vi "solar_addon.vi"(7 "Action (Launch)":enum8{"Launch", "Initialize", "Shutdown"}(ring), 8 "error in (no error)":errorcluster, 9 "SOLAR Refnum":T1, 10 "AddonVIs (Initialize only)":refnum<vi>[](array[refnum]), 11 "Launch Addon VI":string) -> (0 "error out":errorcluster, 3 "Addons (vi,title)":string[][](array[string]))   [LabVIEW 2018]
doc: "This handles the Addon VIs."
uses:
  solar/solar_ctl SOLAR Refnum.ctl
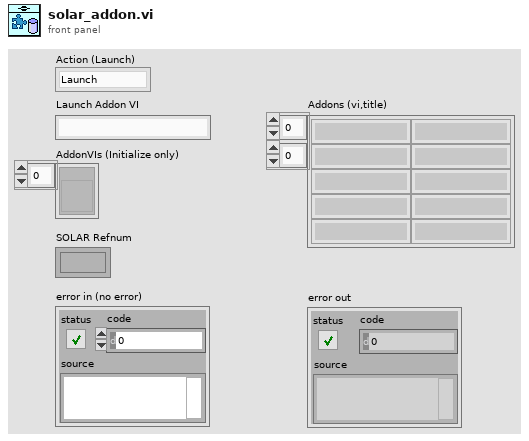
[diagram p1: front panel]
types:
  T1 = typedef "solar_ctl SOLAR Refnum.ctl" = refnum<k1>
  T2 = cluster{"VIName":string, "Title":string, "VI Refnum":refnum<vi>, "Exit":refnum<user-event>}[]
  T3 = cluster{"VIName":string, "Title":string, "VI Refnum":refnum<vi>, "Exit":refnum<user-event>}
  T4 = enum32{"Invalid", "Standard", "Closed", "Hidden", "Minimized", "Maximized"}
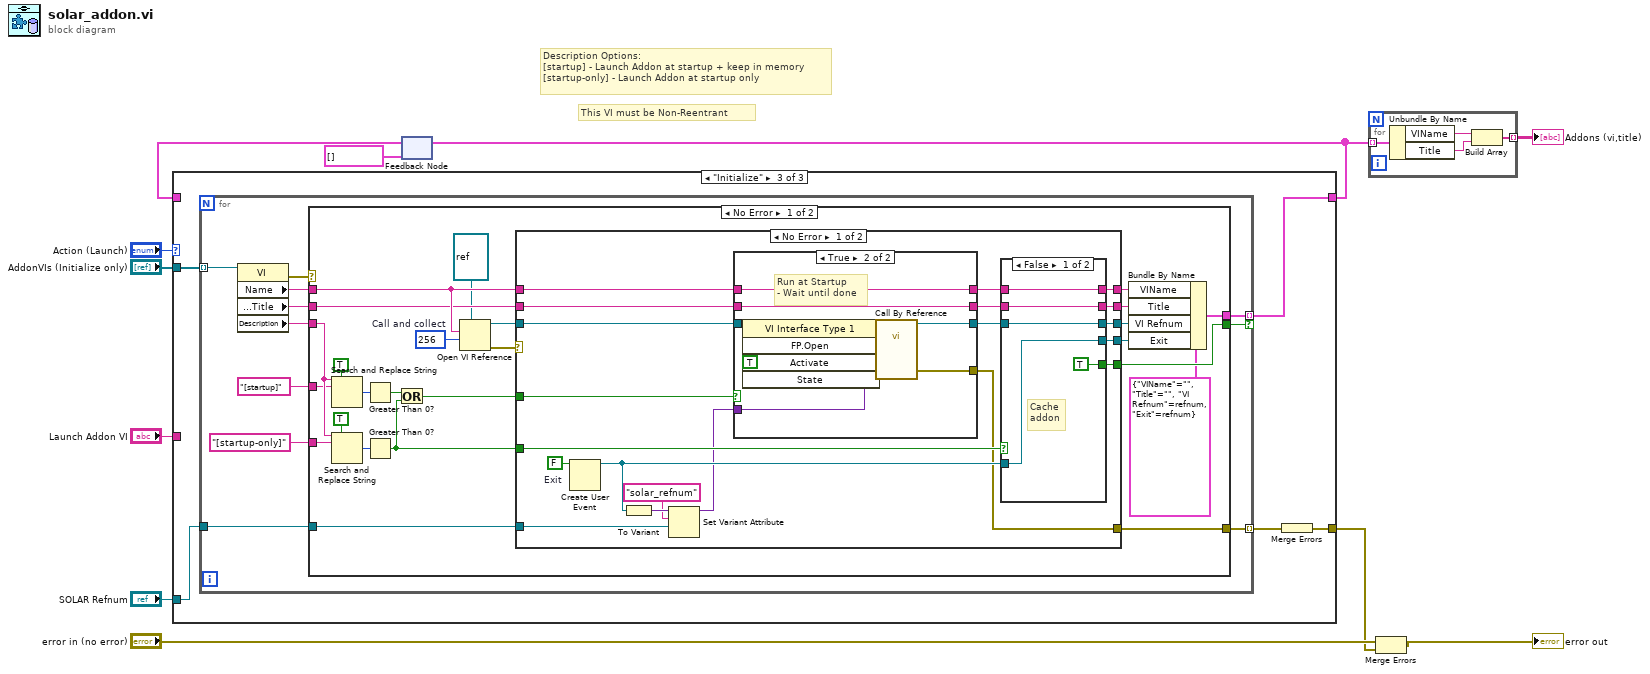
[diagram p0: block diagram]
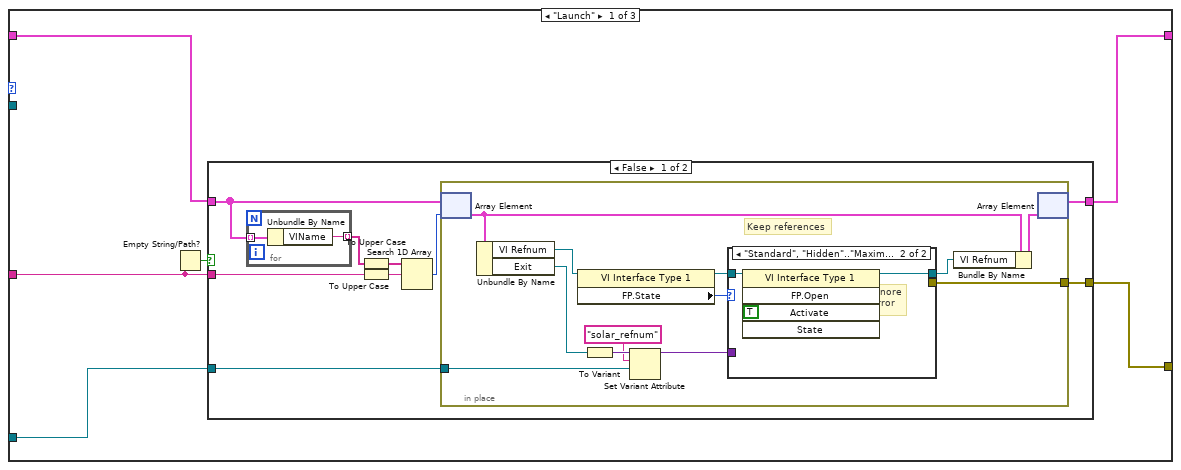
[diagram p2: hidden frame]
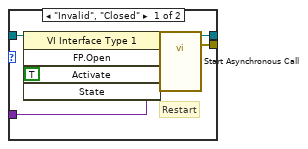
[diagram p3: hidden frame]
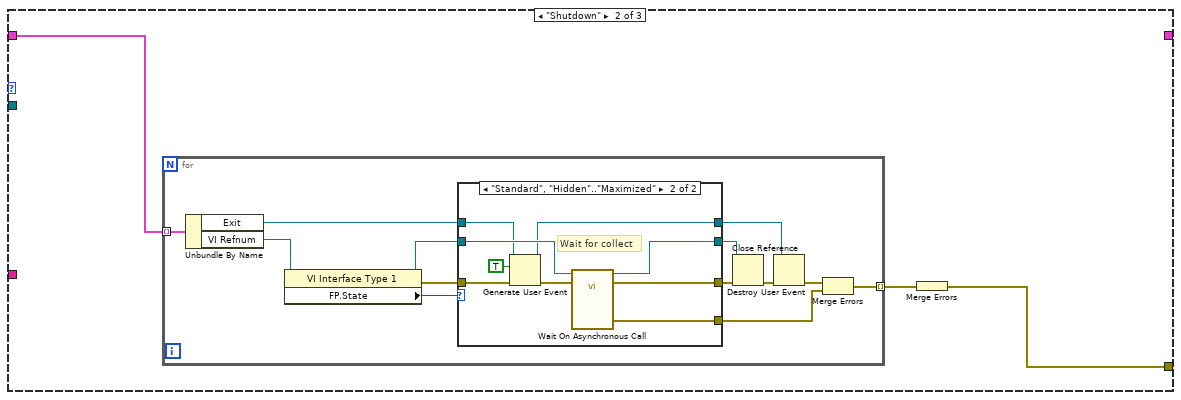
[diagram p5: hidden frame]
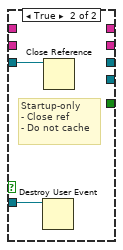
[diagram p7: hidden frame]
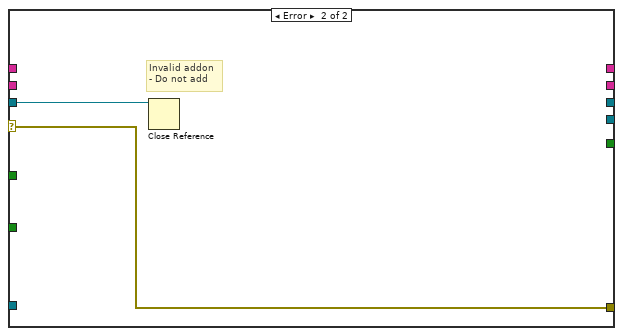
[diagram p9: hidden frame]
diagram:
  # "Description Options:\n[startup] - Launch Addon at startup + keep in memory\n[startup-only] - Launch Addon at startup only"
  # "This VI must be Non-Reentrant"
  n1 = feedback #1(T2 [] ("Array 2")) -> (w4:T2)
  n2 = case shown="\"Initialize\"" "Action (Launch)" {
    tunnel: "AddonVIs (Initialize only)" -> [_ _ w83]
    tunnel: "Launch Addon VI" -> [w17 _ _]
    tunnel: [w13 _ w82] -> w2
    tunnel: w4 -> [w14 w53 _]
    tunnel: "SOLAR Refnum" -> [w12 _ w81]
    tunnel: [w15 w51 w79] -> w3
    frame "Launch" {
      n3 = Empty String/Path?(string/path=w17) -> (empty?=w16:bool)
      n4 = case shown="False" w16 {
        tunnel: w17 -> [w25 _]
        tunnel: w14 -> [w21 w50]
        tunnel: [w22 _] -> w15
        tunnel: [w19 w50] -> w13
        tunnel: w12 -> [w18 _]
        frame False {
          n5 = for {
            tunnel: w21 -> [w49] mode=indexing
            tunnel: [w48] -> w23 mode=indexing
            n6 = Unbundle By Name(w49) -> ("VIName"=w48:string)
          }
          n7 = To Upper Case(1:w23) -> (0:w26:string[])
          n8 = To Upper Case(1:w25) -> (0:w24:string)
          n9 = Search 1D Array(1D array=w26, element=w24) -> (index of element=w20:i32)  [unwired: 1 in]
          n10 = in-place {
            in-place-border: [w38] -> w22
            in-place-border: w18 -> [w29]
            # "Keep references"
            n11 = in-place-array #2(w21, w20) -> (w37:T3)
            n12 = Unbundle By Name(w37) -> ("VI Refnum"=w34:refnum<vi>, "Exit"=w30:refnum<user-event>)
            n13 = property class="VI Interface Type 1"(reference=w34) -> (reference out=w33:refnum<vi>, "FP.State"=w27:T4)  [unwired: 1 in, 1 out]
            n14 = To Variant(anything=w30) -> (Variant=w32:variant)
            n15 = Set Variant Attribute(Variant=w32, name="solar_refnum", value=w29) -> (Variant out=w28:variant)  [unwired: 1 in, 2 out]
            n16 = case shown="\"Standard\", \"Hidden\"..\"Maximized\"" w27 {
              tunnel: [w44 _] -> w38
              tunnel: [w43 w45] -> w35
              tunnel: w33 -> [w41 w46]
              tunnel: w28 -> [w39 _]
              frame "Invalid", "Closed" {
                # "Restart"
                n17 = invoke class="VI Interface Type 1" method="FP.Open"(reference=w41, "Activate"=TRUE ("Activate?")) -> (reference out=w40:refnum<vi>)  [unwired: 3 in, 4 out]
                n18 = call-by-ref "Start Asynchronous Call"(reference=w40, "Variant"=w39) -> (reference out=w43:refnum<vi>, error out=w44:errorcluster)  [unwired: 11 in, 1 out]
              }
              frame "Standard", "Hidden".."Maximized" {
                # "Ignore\nerror"
                n19 = invoke class="VI Interface Type 1" method="FP.Open"(reference=w46, "Activate"=TRUE ("Activate?")) -> (reference out=w45:refnum<vi>)  [unwired: 3 in, 4 out]
              }
            }
            n20 = Bundle By Name(cluster=w37, "VI Refnum"=w35) -> (w36:T3)
            n21 = in-place-array #2(w36) -> (w19:T2)  [unwired: 1 out]
          }
        }
        frame True {
          # "Do nothing"
        }
      }
    }
    frame "Shutdown" {
      n22 = for {
        tunnel: w53 -> [w66] mode=indexing
        tunnel: [w55] -> w52 mode=indexing
        n23 = Unbundle By Name(w66) -> ("Exit"=w63:refnum<user-event>, "VI Refnum"=w62:refnum<vi>)
        n24 = property class="VI Interface Type 1"(reference=w62) -> (reference out=w65:refnum<vi>, error out=w61:errorcluster, "FP.State"=w64:T4)  [unwired: 1 in]
        n25 = case shown="\"Standard\", \"Hidden\"..\"Maximized\"" w64 {
          tunnel: w61 -> [w69 w76]
          tunnel: w65 -> [w68 w78]
          tunnel: w63 -> [w67 w75]
          tunnel: [w69 w72] -> w59
          tunnel: [w68 w73] -> w58
          tunnel: [w67 w71] -> w57
          tunnel: [_ w70] -> w54
          frame "Invalid", "Closed" {
          }
          frame "Standard", "Hidden".."Maximized" {
            # "Wait for collect"
            n26 = Generate User Event(user event=w75, event data cluster=TRUE ("event data"), error in=w76) -> (user event out=w71:refnum<user-event>, error out=w74:errorcluster)  [unwired: 1 in]
            n27 = call-by-ref "Wait On Asynchronous Call"(reference=w78, error in=w74) -> (reference out=w73:refnum<vi>, error out=w72:errorcluster, 0:"error out"=w70:errorcluster)  [unwired: 11 in]
          }
        }
        n28 = Close Reference(reference=w58, error in (no error)=w59) -> (error out=w60:errorcluster)
        n29 = Destroy User Event(user event=w57, error in=w60) -> (error out=w56:errorcluster)
        n30 = Merge Errors(w56, w54) -> (w55:errorcluster)
      }
      n31 = Merge Errors(w52) -> (w51:errorcluster)
    }
    frame "Initialize" {
      n32 = for {
        tunnel: w83 -> [w94] mode=indexing
        tunnel: [w90] -> w82 mode=indexing if=w89
        tunnel: w81 -> [w85]
        tunnel: [w84] -> w80 mode=indexing
        n33 = property class="VI"(reference=w94) -> (error out=w88:errorcluster, "Name"=w92:string, "Front Panel.Title"=w91:string, "Description"=w93:string)  [unwired: 1 in, 1 out]
        n34 = case shown="No Error" w88 {
          selector: w88 -> [_ w160]
          tunnel: w93 -> [w115 _]
          tunnel: w92 -> [w113 _]
          tunnel: w91 -> [w112 _]
          tunnel: [w104 _] -> w90
          tunnel: [w106 _] -> w89
          tunnel: "[startup]" ("search string") -> [w109 _]
          tunnel: "[startup-only]" ("search string") -> [w108 _]
          tunnel: w85 -> [w98 _]
          tunnel: [w95 w160] -> w84
          frame No Error {
            w114 = 256  # Call and collect
            n35 = Search and Replace String(replace all?=TRUE ("replace all? (F)"), input string=w115, search string=w109) -> (number of replacements=w117:i32)  [unwired: 5 in, 3 out]
            n36 = Search and Replace String(replace all?=TRUE ("replace all? (F)"), input string=w115, search string=w108) -> (number of replacements=w118:i32)  [unwired: 5 in, 3 out]
            n37 = Greater Than 0?(x=w117) -> (x > 0?=w110:bool)
            n38 = Greater Than 0?(x=w118) -> (x > 0?=w100:bool)
            n39 = Or(x=w110, y=w100) -> (x .or. y?=w105:bool)
            n40 = Open VI Reference(type specifier VI Refnum (for type only)=refnum<vi> refnum, vi path=w113, options=w114) -> (vi reference=w111:refnum<vi>, error out=w107:errorcluster)  [unwired: 3 in]
            n41 = case shown="No Error" w107 {
              selector: w107 -> [_ w158]
              tunnel: w113 -> [w138 _]
              tunnel: w112 -> [w137 _]
              tunnel: w111 -> [w122 w159]
              tunnel: [w129 _] -> w106
              tunnel: w105 -> [w139 _]
              tunnel: [w135 _] -> w103
              tunnel: [w133 _] -> w102
              tunnel: [w131 _] -> w101
              tunnel: w100 -> [w136 _]
              tunnel: w98 -> [w125 _]
              tunnel: [w123 _] -> w96
              tunnel: [w120 w158] -> w95
              frame No Error {
                w128 = FALSE  # Exit
                n42 = Create User Event(user event datatype=w128) -> (user event=w124:refnum<user-event>)  [unwired: 1 in, 1 out]
                n43 = To Variant(anything=w124) -> (Variant=w127:variant)
                n44 = Set Variant Attribute(Variant=w127, name="solar_refnum", value=w125) -> (Variant out=w121:variant)  [unwired: 1 in, 2 out]
                n45 = case shown="True" w139 {
                  tunnel: w122 -> [w147 w156]
                  tunnel: [w147 w152] -> w130
                  tunnel: [w149 w155] -> w134
                  tunnel: w138 -> [w149 w155]
                  tunnel: w137 -> [w148 w154]
                  tunnel: [w148 w154] -> w132
                  tunnel: w121 -> [_ w151]
                  tunnel: [_ w150] -> w120
                  frame False {
                  }
                  frame True {
                    # "Run at Startup\n- Wait until done"
                    n46 = invoke class="VI Interface Type 1" method="FP.Open"(reference=w156, "Activate"=TRUE ("Activate?")) -> (reference out=w153:refnum<vi>)  [unwired: 3 in, 4 out]
                    n47 = call-by-ref "?"(reference=w153, "Variant"=w151) -> (reference out=w152:refnum<vi>, "error out"=w150:errorcluster)  [unwired: 11 in, 1 out]
                  }
                }
                n48 = case shown="False" w136 {
                  tunnel: [w144 _] -> w135
                  tunnel: w134 -> [w144 _]
                  tunnel: [w143 _] -> w133
                  tunnel: w132 -> [w143 _]
                  tunnel: [w142 _] -> w131
                  tunnel: w130 -> [w142 w146]
                  tunnel: [TRUE _] -> w129
                  tunnel: w124 -> [w140 w145]
                  tunnel: [w140 _] -> w123
                  frame False {
                    # "Cache\naddon"
                  }
                  frame True {
                    # "Startup-only\n- Close ref\n- Do not cache"
                    n49 = Destroy User Event(user event=w145) -> ()  [unwired: 1 in, 1 out]
                    n50 = Close Reference(reference=w146) -> ()  [unwired: 1 in, 1 out]
                  }
                }
              }
              frame Error {
                # "Invalid addon\n- Do not add"
                n51 = Close Reference(reference=w159) -> ()  [unwired: 1 in, 1 out]
              }
            }
            n52 = Bundle By Name(cluster=T3 {"VIName"="", "Title"="", "VI Refnum"=refnum, "Exit"=refnum} ("Addon"), "VIName"=w103, "Title"=w102, "VI Refnum"=w101, "Exit"=w96) -> (w104:T3)
          }
          frame Error {
          }
        }
      }
      n53 = Merge Errors(w80) -> (w79:errorcluster)
    }
  }
  n54 = feedback-in #1(w2) -> ()
  n55 = for {
    tunnel: w2 -> [w164] mode=indexing
    tunnel: [w161] -> w7 mode=indexing
    n56 = Unbundle By Name(w164) -> ("VIName"=w163:string, "Title"=w162:string)
    n57 = Build Array(w163, w162) -> (w161:string[])
  }
  "Addons (vi,title)" <- w7
  n58 = Merge Errors("error in (no error)", w3) -> (→"error out":errorcluster)
